vi "TestPurePursuit.vi"() -> ()   [LabVIEW 2017]
panel:
  out "Waveform Chart 2":cluster{"LeftValue":dbl, "RightValue":dbl}(graph)
  out "Waveform Chart":dbl(graph)
  in  "Gains":T1={"FFV"=0.0088, "FFA"=0.0017, "Vel PID"={"P"=0.02, "I"=0.0, "D"=0.0}} {"Vel PID"."D" format="%.5f"; "Vel PID"."I" format="%.3f"; "Vel PID"."P" format="%.3f"}
  out "Graph":cluster{cluster{"x":dbl, "y":dbl}[]}[](graph)=[{[{"x"=0.0, "y"=0.0}, {"x"=5.995246383338454, "y"=-0.004012645828084032}, {"x"=11.989963709165476, "y"=-0.008468417857639667}, {"x"=17.98354297984351, "y"=-0.013889086205739646}, {"x"=23.975271652913907, "y"=-0.020878472376735895}, {"x"=29.964243956597706, "y"=-0.030196746534612535}, {"x"=35.94924430892478, "y"=-0.04286620444492253}, {"x"=41.928610635591134, "y"=-0.06029035080001573}, {"x"=47.9000545251606, "y"=-0.08440348886793915}, {"x"=53.86040660212064, "y"=-0.11788275539924309}, {"x"=59.805260034137504, "y"=-0.16444975200463963}, {"x"=65.72847725734516, "y"=-0.2292854981121004}, {"x"=71.62152260700609, "y"=-0.31960508446336955}, {"x"=77.4724866556623, "y"=-0.44545539796388384}, {"x"=83.26484875329494, "y"=-0.6208031514378805}, {"x"=88.97549654447519, "y"=-0.8651537401081744}, {"x"=94.57232171382118, "y"=-1.205619932505254}, {"x"=100.01053645428007, "y"=-1.6800275219578666}, {"x"=105.22769885621243, "y"=-2.341106494164938}, {"x"=110.13683343978134, "y"=-3.262294268149245}, {"x"=114.61673554465331, "y"=-4.545956287431122}, {"x"=118.49851472810515, "y"=-6.334705246910349}, {"x"=121.54678812252946, "y"=-8.827319936613026}, {"x"=123.65580321621499, "y"=-12.300761597955725}, {"x"=125.09320280597504, "y"=-16.475113357990896}, {"x"=126.05199193535013, "y"=-21.148356536761245}, {"x"=126.67198454498464, "y"=-26.173918530995163}, {"x"=127.0553578248398, "y"=-31.444362449889}, {"x"=127.27800699667785, "y"=-36.87944955235837}, {"x"=127.39796774339639, "y"=-42.41723767588606}, {"x"=127.46186036667065, "y"=-48.00720340057727}, {"x"=127.5100734436229, "y"=-53.6046228218006}, {"x"=127.58125458910263, "y"=-59.16559779997397}, {"x"=127.71660386470693, "y"=-64.64217947366461}, {"x"=127.96445005632496, "y"=-69.97704309012738}, {"x"=128.38562122946817, "y"=-75.09711843149461}, {"x"=129.0602053715568, "y"=-79.90546877696795}, {"x"=130.09644976298665, "y"=-84.27051900515752}, {"x"=131.64278708257433, "y"=-88.01143722629587}, {"x"=133.90432586141884, "y"=-90.87804434065568}, {"x"=137.15523551566062, "y"=-92.73109962945875}, {"x"=141.09676030370667, "y"=-93.87077976674169}, {"x"=145.50687993024508, "y"=-94.51799922038093}, {"x"=150.21564224442068, "y"=-94.83894924101895}, {"x"=155.08627613061006, "y"=-94.96357484257668}, {"x"=160.0, "y"=-95.0}]}, {[{"x"=162.61719179857315, "y"=-94.24442448910123}, {"x"=174.2188679085159, "y"=-91.17830129523192}]}, {[{"x"=145.50687993024508, "y"=-94.51799922038093}]}, {[{"x"=177.61719179857315, "y"=-94.24442448910123}, {"x"=174.75244671419736, "y"=-85.42764570471414}, {"x"=167.25244671419736, "y"=-79.97857674467393}, {"x"=157.98193688294893, "y"=-79.97857674467393}, {"x"=150.48193688294893, "y"=-85.42764570471414}, {"x"=147.61719179857315, "y"=-94.24442448910123}, {"x"=150.48193688294893, "y"=-103.06120327348833}, {"x"=157.98193688294893, "y"=-108.51027223352854}, {"x"=167.25244671419736, "y"=-108.51027223352854}, {"x"=174.75244671419736, "y"=-103.06120327348833}, {"x"=177.61719179857315, "y"=-94.24442448910123}]}, {[{"x"=128.2290009515077, "y"=-67.7637799941129}, {"x"=133.45998967618738, "y"=-83.86310787520901}, {"x"=147.15489595216633, "y"=-93.81303970175523}, {"x"=164.0827310547648, "y"=-93.81303970175523}, {"x"=177.77763733074374, "y"=-83.86310787520901}, {"x"=183.00862605542343, "y"=-67.7637799941129}, {"x"=177.77763733074374, "y"=-51.66445211301679}, {"x"=164.0827310547648, "y"=-41.71452028647057}, {"x"=147.15489595216633, "y"=-41.71452028647056}, {"x"=133.45998967618738, "y"=-51.66445211301678}, {"x"=128.2290009515077, "y"=-67.7637799941129}]}]
  in  "Max Accel":dbl=50.0 format="%#_13g"
  in  "MaxVel":dbl(slide)=100.0 scale=0.0..100.0
  in  "LookAhead":dbl=15.0
  in  "Path":cluster{"x":dbl, "y":dbl}[](array[cluster])=[{"x"=0.0, "y"=0.0}, {"x"=130.0, "y"=0.0}, {"x"=125.0, "y"=-100.0}, {"x"=160.0, "y"=-95.0}]
  in  "Config":T2={"Gear Reduction"=15.0, "Wheel Radius (m)"=0.076, "# Motors"=1, "coeff of friction"=0.1, "Mass (kg)"=50.0, "Motor"={"Ke (V)"=0.0183, "R (ohms)"=0.09, "KT (Nm/A)"=0.0183, "Tf (Nm)"=0.4}}
  # ".007"
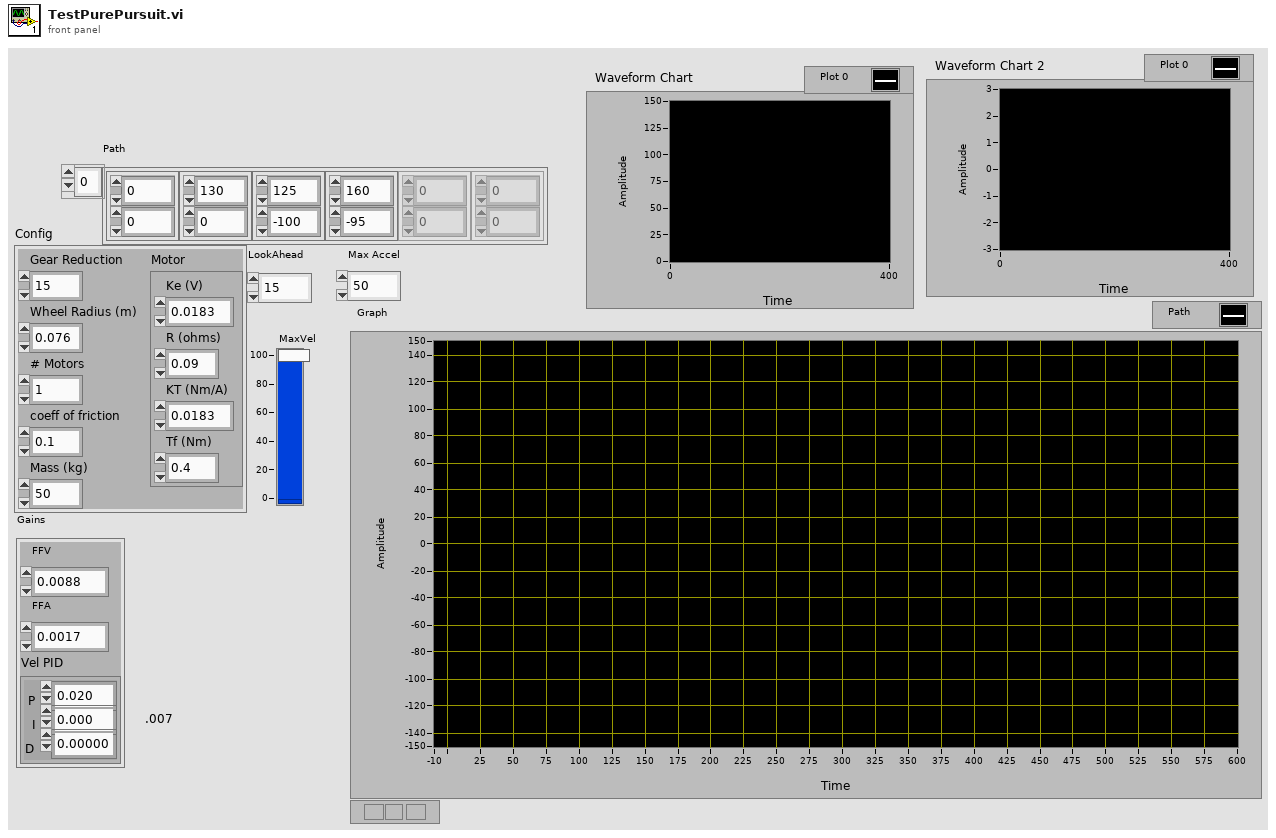
[diagram p1: front panel]
types:
  T1 = cluster{"FFV":dbl, "FFA":dbl, "Vel PID":cluster{"P":dbl, "I":dbl, "D":dbl}}
  T2 = cluster{"Gear Reduction":dbl, "Wheel Radius (m)":dbl, "# Motors":u32, "coeff of friction":dbl, "Mass (kg)":dbl, "Motor":cluster{"Ke (V)":dbl, "R (ohms)":dbl, "KT (Nm/A)":dbl, "Tf (Nm)":dbl}}
  T3 = cluster{"SmoothPath":cluster{dbl, dbl}[], "Distance":dbl}
  T4 = cluster{"LeftDistance":dbl, "RightDistance":dbl, "LeftVelocity":dbl, "RightVelocity":dbl, "Angle":dbl, "Location":cluster{dbl, dbl}}
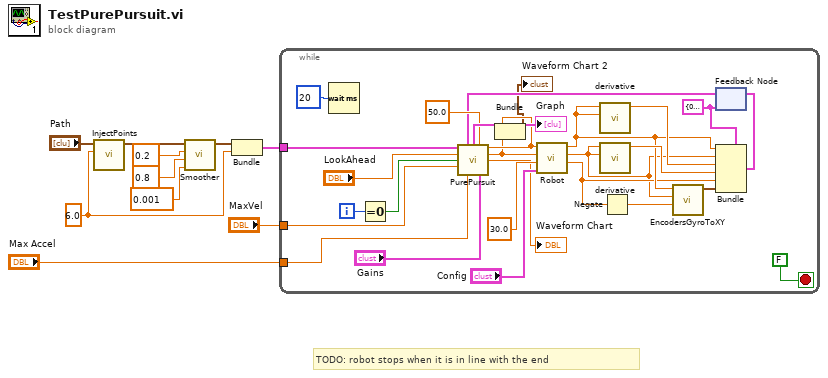
[diagram p0: block diagram]
diagram:
  w6 = 6.0 ("Distance")
  # "TODO: robot stops when it is in line with the end"
  n1 = call "InjectPoints.vi"("Spacing"=w6, "Path"="Path") -> ("Path out"=w4:cluster{dbl, dbl}[])  [unwired: 9 in]
  n2 = call "Smoother.vi"("tolerance"=0.001, "B"=0.8, "A"=0.2, "Path"=w4) -> ("SmoothPath"=w1:cluster{dbl, dbl}[])  [unwired: 7 in]
  n3 = Bundle("SmoothPath"=w1, "Distance"=w6) -> (w5:T3)  [unwired: 1 in]
  n4 = while {
    tunnel: w5 -> [w18]
    tunnel: "MaxVel" -> [w17]
    tunnel: "Max Accel" -> [w16]
    i -> [w15]
    stop <- FALSE stop-if-true
    w27 = T4 {"LeftDistance"=0.0, "RightDistance"=0.0, "LeftVelocity"=0.0, "RightVelocity"=0.0, "Angle"=0.0, "Location"={0.0, 0.0}} ("SensorData")
    n5 = Wait (ms)(milliseconds to wait=u32 20) -> ()  [unwired: 1 out]
    n6 = Equal To 0?(x=w15) -> (x = 0?=w14:bool)
    n7 = feedback #1(w27) -> (w21:T4)
    n8 = call "PurePursuit.vi"("PathData"=w18, "SensorData"=w21, "Trackwidth"=50.0, "LookAhead"="LookAhead", "Reset"=w14, "MaxVel"=w17, "Max Accel"=w16, "Gains"="Gains") -> ("Graph"=→"Graph":cluster{cluster{"x":dbl, "y":dbl}[]}[], "LeftValue"=w13:dbl, "RightValue"=w12:dbl, "TargetVel"=→"Waveform Chart":dbl)  [unwired: 3 in, 1 out]
    n9 = Bundle("LeftValue"=w13, "RightValue"=w12) -> (→"Waveform Chart 2":cluster{"LeftValue":dbl, "RightValue":dbl})  [unwired: 1 in]
    n10 = call "Robot.vi"("Config"="Config", "WheelBase"=30.0, "Right Value"=w12, "Left Value"=w13) -> ("Angle"=w20:dbl, "Right Distance"=w19:dbl, "Left Distance"=w24:dbl)  [unwired: 5 in]
    n11 = call "derivative.vi"("Starting value"=w24, "x"=w24) -> ("dx/dt"=w26:dbl)  [unwired: 9 in]
    n12 = call "derivative.vi"("Starting value"=w19, "x"=w19) -> ("dx/dt"=w25:dbl)  [unwired: 9 in]
    n13 = Negate(x=w20) -> (-x=w23:dbl)
    n14 = call "EncodersGyroToXY.vi"("Angle (degrees)"=w23, "Right Distance"=w19, "Left Distance"=w24) -> ("Location"=w22:cluster{dbl, dbl})  [unwired: 8 in]
    n15 = Bundle(cluster=w27, "LeftDistance"=w24, "RightDistance"=w19, "LeftVelocity"=w26, "RightVelocity"=w25, "Angle"=w20, "Location"=w22) -> (w33:T4)
    n16 = feedback-in #1(w33) -> ()
  }
